vi "Do Core.vi"(8 "error in (no error)":errorcluster, 9 "Actor in":refnum<class "Actor.lvclass">, 11 "Reply Message":refnum<class "Replay Cmd Msg.lvclass">) -> (0 "error out":errorcluster, 1 "Actor out":refnum<class "Actor.lvclass">, 2 "Reply":variant)   [LabVIEW 2020, in "Generic Actor.lvlib" / "Replay Cmd Msg.lvclass"]
doc: "(<B>Filename</B>: Actor Framework.lvlib:Reply Msg.lvclass:Do Core.vi)\n\nDefines what an actor does when it receives <B>Reply Message</B>. This method also defines the <B>Reply</B> that is returned to the actor that sent <B>Reply Message</B>.\n\nBy default, this method does nothing, and <B>Reply</B> is the ancestor Message class. A child class must override this method to define behavior and specify a child of the Message class to return in the <B>Reply</B> output."
uses:
  Replay Cmd Msg.lvclass
  <vilib>/ActorFramework/Actor/Actor.lvclass
  Generic Actor/Generic Actor.lvclass
  C:/Program Files (x86)/National Instruments/LabVIEW 2020/vi.lib/ActorFramework/Actor/Actor.lvclass
  Replay Cmd Msg.lvclass/Replay Cmd Msg.ctl
  98bd18b0-b084-4b01-8892-99e7cff396cc.vi
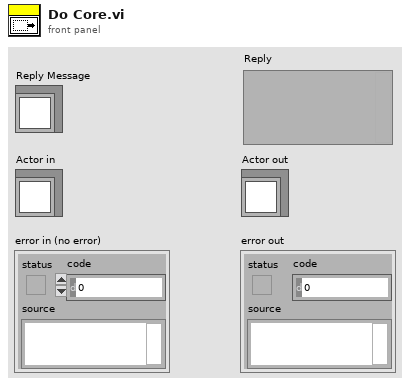
[diagram p1: front panel]
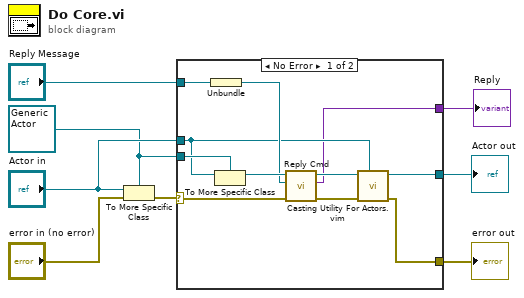
[diagram p0: block diagram]
diagram:
  w5 = refnum<class "Generic Actor.lvclass"> refnum ("Generic Actor.lvlib:Generic Actor.lvclass")
  n1 = To More Specific Class(target class=w5, reference="Actor in", error in="error in (no error)") -> (error out=w7:errorcluster)  [unwired: 1 out]
  n2 = case shown="No Error" w7 {
    selector: w7 -> [w17 w20]
    tunnel: "Actor in" -> [w11 w21]
    tunnel: w5 -> [w19 _]
    tunnel: "Reply Message" -> [w16 _]
    tunnel: [w13 w20] -> w3
    tunnel: [w10 w21] -> w2
    tunnel: [w9 _] -> w1
    frame No Error {
      n3 = Unbundle(w16) -> (w15:refnum<class "Generic Cmd.lvclass">)
      n4 = To More Specific Class(target class=w19, reference=w11) -> (specific class reference=w18:refnum<class "Generic Actor.lvclass">)  [unwired: 1 in, 1 out]
      n5 = call-dynamic "Reply Cmd.vi"("error in (no error)"=w17, "Cmd"=w15, "Generic Actor in"=w18) -> ("error out"=w14:errorcluster, "Reply"=w9:variant, "Generic Actor out"=w12:refnum<class "Generic Actor.lvclass">)  [unwired: 6 in]
      n6 = call "Casting Utility For Actors.vim"("type"=w11, "error in (no error)"=w14, "Actor in"=w12) -> ("error out"=w13:errorcluster, "Actor out"=w10:refnum<class "Actor.lvclass">)  [unwired: 7 in]
    }
    frame Error {
    }
  }
  "error out" <- w3
  "Actor out" <- w2
  "Reply" <- w1
